vi "control maju mudur.vi"() -> ()   [LabVIEW 2016]
uses:
  <vilib>/Utility/error.llb/Error Cluster From Error Code.vi
  <vilib>/myRIO/Common/Instrument Driver Framework/myRIO v1.0/PWM/vis/myRIO v1.0 Write PWM.vi
  <vilib>/myRIO/Instrument Drivers/Onboard IO/PWM/PWM.lvlib
panel:
  in  "RF":tag
  in  "RB":tag
  in  "LB":tag
  in  "LF":tag
  in  "dutcy":dbl(slide) scale=0.0..1.0
  in  "Frequency [Hz]":dbl
  in  "stop":bool
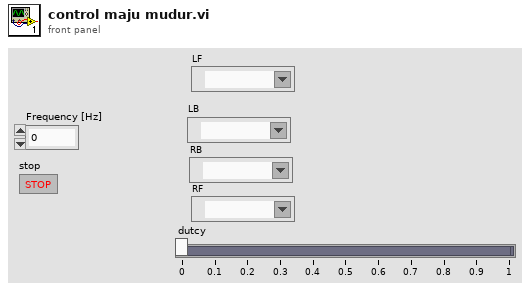
[diagram p1: front panel]
types:
  T1 = typedef "PWM.lvlib/PWM Reference.ctl" = cluster{"myRIO Reference":T2, "PWM Channels Enum":T6, "PWM Configuration":T7}
  T2 = typedef "myRIO Generic Hardware Reference.ctl" = cluster{"myRIO Model":T3, "myRIO Hardware Reference":T4}
  T3 = typedef "Hardware Version Enum.ctl" = enum16{"Unknown", "myRIO-1900", "myRIO-1950", "roboRIO", "NI ELVIS RIO CM"}
  T4 = typedef "myRIO v1.0 Reference.ctl" = cluster{"Generic FPGA Reference":T5, "Allow multiple opens":bool}
  T5 = typedef "Generic FPGA Reference.ctl" = refnum<k20>
  T6 = typedef "PWM Channels Enum.ctl" = enum16{"Not Connected", "C/PWM0", "C/PWM1", "A/PWM0", "A/PWM1", "A/PWM2", "B/PWM0", "B/PWM1", "B/PWM2", "PWM/PWM0", "PWM/PWM1", "PWM/PWM2", "PWM/PWM3", "PWM/PWM4", "PWM/PWM5", "PWM/PWM6", "PWM/PWM7", "PWM/PWM8", "PWM/PWM9"}
  T7 = typedef "PWM.lvlib/PWM Configuration.ctl" = cluster{"Frequency":dbl, "Duty Cycle":dbl}
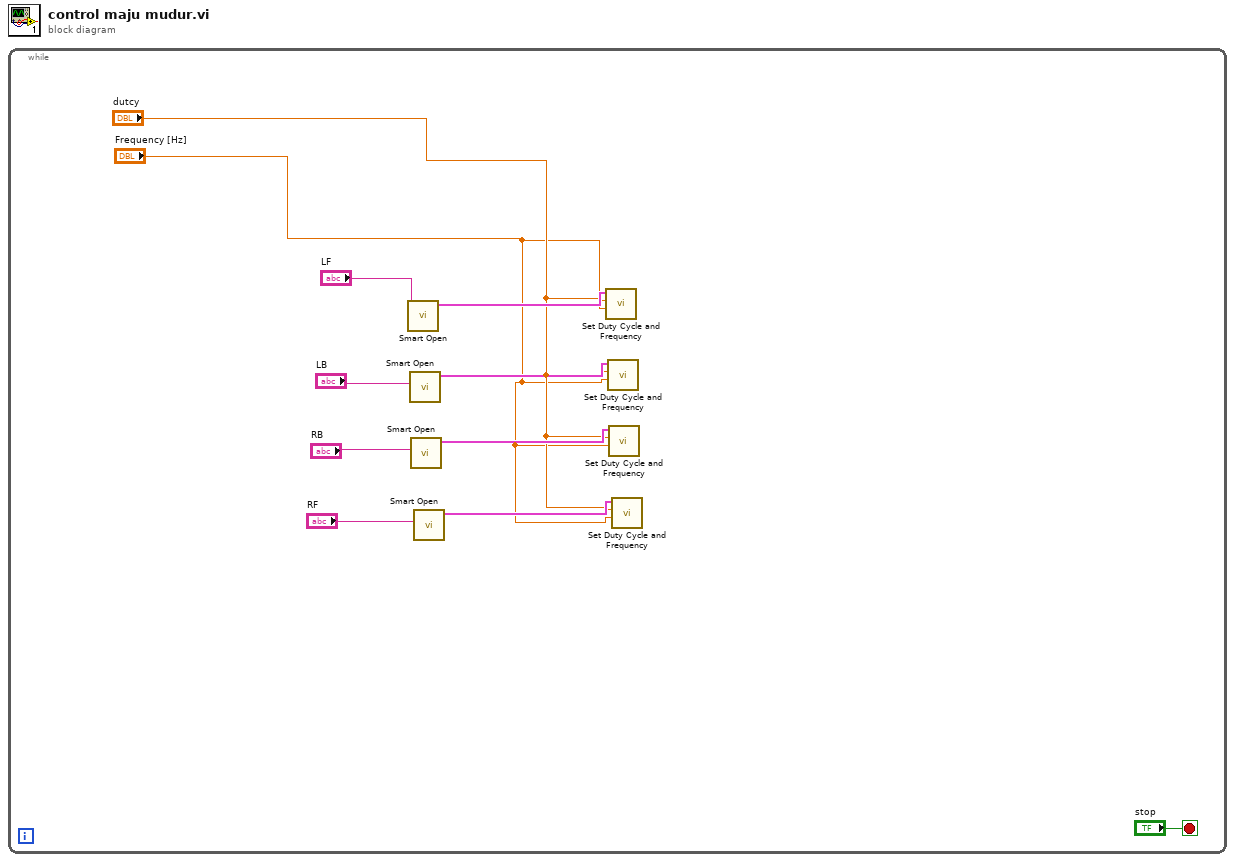
[diagram p0: block diagram]
diagram:
  n1 = while {
    stop <- "stop" stop-if-true
    n2 = call <vilib>:"Smart Open.vi"("Channel Name"="LF") -> ("PWM Ref Out"=w10:T1)  [unwired: 9 in, 1 out]
    n3 = call <vilib>:"Smart Open.vi"("Channel Name"="LB") -> ("PWM Ref Out"=w9:T1)  [unwired: 9 in, 1 out]
    n4 = call <vilib>:"Smart Open.vi"("Channel Name"="RB") -> ("PWM Ref Out"=w8:T1)  [unwired: 9 in, 1 out]
    n5 = call <vilib>:"Smart Open.vi"("Channel Name"="RF") -> ("PWM Ref Out"=w7:T1)  [unwired: 9 in, 1 out]
    n6 = call <vilib>:"Set Duty Cycle and Frequency.vi"("Frequency [Hz]"="Frequency [Hz]", "Duty Cycle"="dutcy", "PWM Ref In"=w10) -> ()  [unwired: 6 in, 2 out]
    n7 = call <vilib>:"Set Duty Cycle and Frequency.vi"("Frequency [Hz]"="Frequency [Hz]", "Duty Cycle"="dutcy", "PWM Ref In"=w9) -> ()  [unwired: 6 in, 2 out]
    n8 = call <vilib>:"Set Duty Cycle and Frequency.vi"("Frequency [Hz]"="Frequency [Hz]", "Duty Cycle"="dutcy", "PWM Ref In"=w8) -> ()  [unwired: 6 in, 2 out]
    n9 = call <vilib>:"Set Duty Cycle and Frequency.vi"("Frequency [Hz]"="Frequency [Hz]", "Duty Cycle"="dutcy", "PWM Ref In"=w7) -> ()  [unwired: 6 in, 2 out]
  }
